vi "SDSU_OpenLib.vi"(8 "error in (no error)":errorcluster, 10 "libdir":path=path "/home/bonati/panview_current/PAN/Modules/SDSU/private/c/lib") -> (0 "error out":errorcluster, 2 "msg out":string)   [LabVIEW 2016]
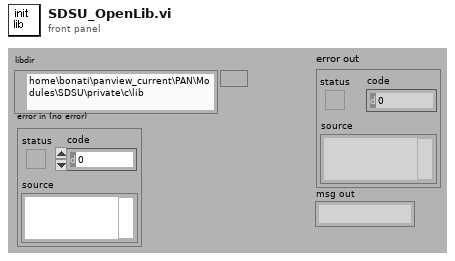
[diagram p1: front panel]
types:
  T1 = enum16{"get fd", "set fd", "add ", "set_readtime", "get all", "clean all", "get by fd"}
  T2 = typedef "DHE_Device.ctl" = cluster{"DevNo":i32, "fd":i32, "name":string, "FPA":string, "modifiers":string, "binpatt":string, "readtime":dbl, "readmode":string, "type":string, "params":string}
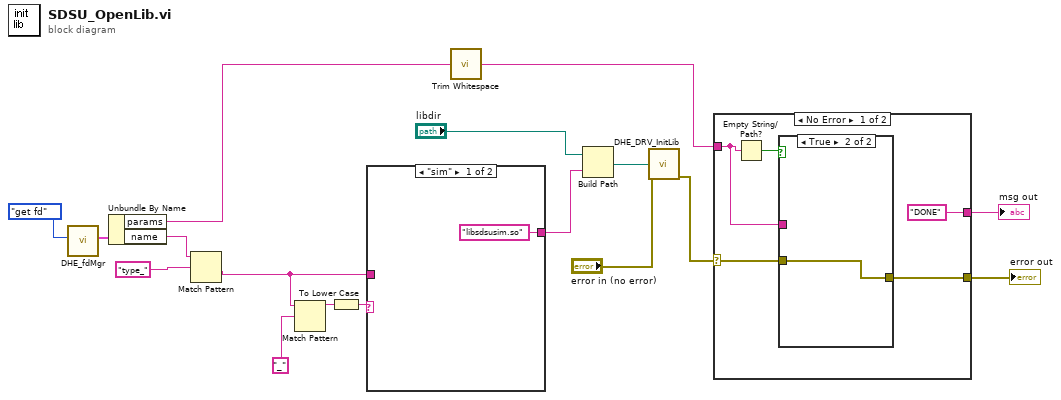
[diagram p0: block diagram]
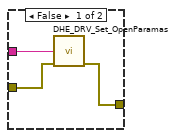
[diagram p2: hidden frame]
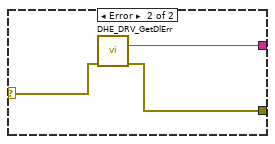
[diagram p3: hidden frame]
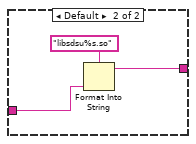
[diagram p4: hidden frame]
diagram:
  n1 = call "DHE_fdMgr.vi"("action"=T1."get fd") -> ("Device"=w16:T2)  [unwired: 4 in, 6 out]
  n2 = Unbundle By Name(w16) -> ("params"=w6:string, "name"=w1:string)
  n3 = Match Pattern(string=w1, regular expression="type_") -> (after substring=w2:string)  [unwired: 4 out]
  n4 = Match Pattern(string=w2, regular expression="_") -> (before substring=w13:string)  [unwired: 4 out]
  n5 = To Lower Case(string=w13) -> (all lower case string=w12:string)
  n6 = case shown="\"sim\"" w12 {
    tunnel: w2 -> [_ w20]
    tunnel: ["libsdsusim.so" w19] -> w10
    frame "sim" {
    }
    frame Default {
      n7 = Format Into String(format string="libsdsu%s.so", w20) -> (resulting string=w19:string)  [unwired: 2 in, 1 out]
    }
  }
  n8 = call <vilib>:"Trim Whitespace.vi"("string"=w6) -> ("trimmed string"=w5:string)  [unwired: 1 in]
  n9 = Build Path(base path="libdir", name or relative path=w10) -> (appended path=w9:path)
  n10 = call "DHE_DRV_InitLib.vi"("filepath"=w9, "error in (no error)"="error in (no error)") -> ("error out"=w7:errorcluster)  [unwired: 13 out]
  n11 = case shown="No Error" w7 {
    selector: w7 -> [w24 w33]
    tunnel: w5 -> [w25 _]
    tunnel: [w23 w32] -> w4
    tunnel: ["DONE" ("err out") w31] -> w3
    frame No Error {
      n12 = Empty String/Path?(string/path=w25) -> (empty?=w26:bool)
      n13 = case shown="True" w26 {
        tunnel: w25 -> [w29 _]
        tunnel: w24 -> [w28 w30]
        tunnel: [w27 w30] -> w23
        frame False {
          n14 = call "DHE_DRV_Set_OpenParamas.vi"("params"=w29, "error in (no error)"=w28) -> ("error out"=w27:errorcluster)  [unwired: 13 out]
        }
        frame True {
        }
      }
    }
    frame Error {
      n15 = call "DHE_DRV_GetDlErr.vi"("error in (no error)"=w33) -> ("err out"=w31:string, "error out"=w32:errorcluster)  [unwired: 13 out]
    }
  }
  "error out" <- w4
  "msg out" <- w3
